vi "Obtain Control Cluster.vi"(9 "I/O":bool=TRUE, 10 "Dispense":bool=TRUE, 11 "Motion":bool=TRUE) -> (3 "Control Out":T1)   [LabVIEW 2016, in "Controller.lvclass"]
uses:
  Controller.lvclass
  Controllers.ctl
  Motion/Motion Folder/Motion.lvclass
  I-O/I-O Folder/I-O.lvclass
  Dispenser/Dispenser Folder/Dispenser.lvclass
  Dispenser/Ultimus V2 Folder/Ultimus V2.lvclass
  D:/Gantry_General/Classes/Controller/Dispenser/Dispenser Folder/Dispenser.lvclass
  Motion/A3200 Folder/A3200.lvclass
  D:/Gantry_General/Classes/Controller/Motion/Motion Folder/Motion.lvclass
  I-O/NI-DAQ Folder/NI-DAQ.lvclass
  D:/Gantry_General/Classes/Controller/I-O/I-O Folder/I-O.lvclass
panel:
  in  "Control":T1
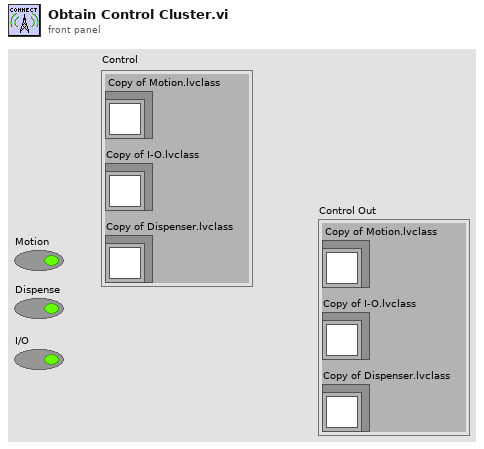
[diagram p1: front panel]
types:
  T1 = typedef "Controller.lvclass/Controllers.ctl" = cluster{"Copy of Motion.lvclass":refnum<class "Motion.lvclass">, "Copy of I-O.lvclass ":refnum<class "I-O.lvclass">, "Copy of Dispenser.lvclass":refnum<class "Dispenser.lvclass">}
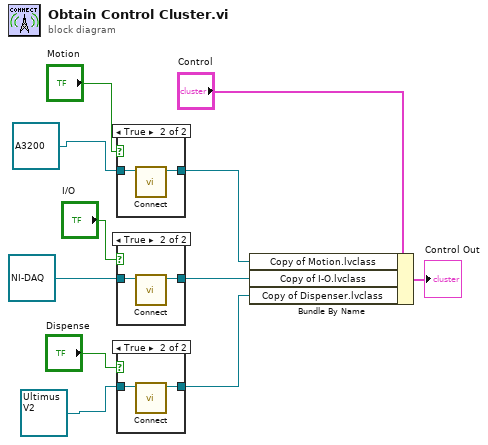
[diagram p0: block diagram]
diagram:
  n1 = case shown="True" "Motion" {
    tunnel: [w12 w13] -> w6
    tunnel: refnum<class "A3200.lvclass"> refnum ("A3200.lvclass") -> [w12 w14]
    frame False {
    }
    frame True {
      n2 = call-dynamic "Connect.vi"("Gantry in"=w14) -> ("Gantry out"=w13:refnum<class "A3200.lvclass">)  [unwired: 9 in, 1 out]
    }
  }
  n3 = case shown="True" "I/O" {
    tunnel: refnum<class "NI-DAQ.lvclass"> refnum ("NI-DAQ.lvclass") -> [w15 w17]
    tunnel: [w15 w16] -> w5
    frame False {
    }
    frame True {
      n4 = call-dynamic "Connect.vi"("NI-DAQ in"=w17) -> ("NI-DAQ out"=w16:refnum<class "NI-DAQ.lvclass">)  [unwired: 9 in, 1 out]
    }
  }
  n5 = case shown="True" "Dispense" {
    tunnel: refnum<class "Ultimus V2.lvclass"> refnum ("Ultimus V2.lvclass") -> [w18 w20]
    tunnel: [w18 w19] -> w4
    frame False {
    }
    frame True {
      n6 = call-dynamic "Connect.vi"("Ultimus V in"=w20) -> ("Ultimus V out"=w19:refnum<class "Ultimus V2.lvclass">)  [unwired: 9 in, 1 out]
    }
  }
  n7 = Bundle By Name(cluster="Control", "Copy of Motion.lvclass"=w6, "Copy of I-O.lvclass"=w5, "Copy of Dispenser.lvclass"=w4) -> (→"Control Out":T1)
